vi "Write $GPRMC.vi"(8 "error in (no error)":errorcluster, 10 "GPRMC-data":T1={"TimeStamp"=timestamp(0 s since 1904-01-01), "Validity"=FALSE, "Latitude"=0.0, "Latitude-Direction"=enum."North", "Longitude"=0.0, "Longitude-Direction"=enum."East", "Speed in knots"=0.0, "True course"=0.0, "Date Stamp"=timestamp(0 s since 1904-01-01), "Magnetic Variation (East/West)"=0.0, "GPS Latitude"=0.0, "GPS Longitude"=0.0} {"GPS Longitude" format="%.6f"; "GPS Latitude" format="%.6f"; "Magnetic Variation (East/West)" format="%.02f [deg]"; "Date Stamp" format="%<%x>T"; "True course" format="%.02f [deg]"; "Speed in knots" format="%.02f [kts]"; "Longitude" format="%0.4f [long]"; "Latitude" format="%.04f [lat]"; "TimeStamp" format="%<%.2X>T"}, 11 "GPS Data Message in":refnum<class "GPS Data Message.lvclass">) -> (0 "error out":errorcluster, 3 "GPS Data Message out":refnum<class "GPS Data Message.lvclass">)   [LabVIEW 2015, in "RDS Child Messages.lvlib" / "GPS Data Message.lvclass"]
uses:
  GPS Data Message.lvclass
  3rd Party/NMEA_GPS/NMEA_GPRMC-data.ctl
  3rd Party/NMEA_GPS/NMEA_LatitudeDirection.ctl
  3rd Party/NMEA_GPS/NMEA_LongitudeDirection.ctl
  GPS Data Message.lvclass/GPS Data Message.ctl
  3rd Party/NMEA_GPS/NMEA.lvlib
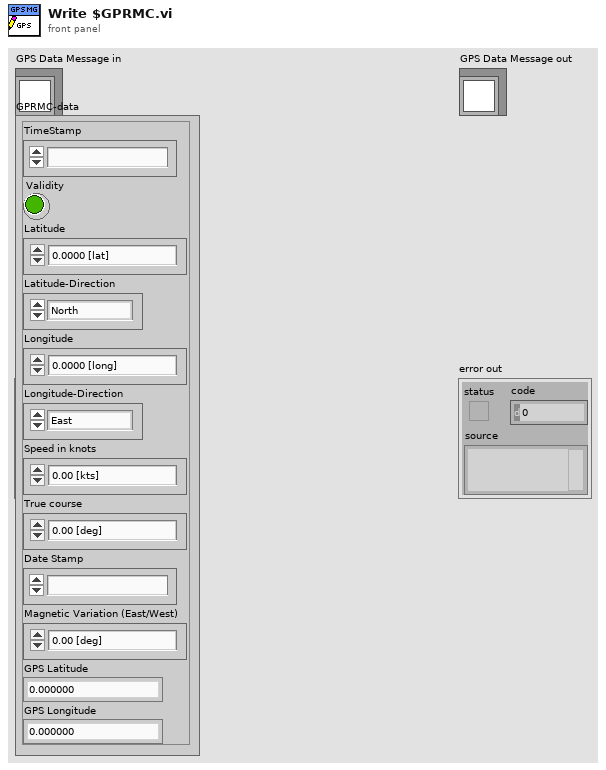
[diagram p1: front panel]
types:
  T1 = typedef "RDS Libraries.lvlib/NMEA.lvlib/NMEA_GPRMC-data.ctl" = cluster{"TimeStamp":timestamp, "Validity":bool, "Latitude":dbl, "Latitude-Direction":T2, "Longitude":dbl, "Longitude-Direction":T3, "Speed in knots":sgl, "True course":sgl, "Date Stamp":timestamp, "Magnetic Variation (East/West)":sgl, "GPS Latitude":dbl, "GPS Longitude":dbl}
  T2 = typedef "RDS Libraries.lvlib/NMEA.lvlib/NMEA_LatitudeDirection.ctl" = enum16{"", "North", "South"}
  T3 = typedef "RDS Libraries.lvlib/NMEA.lvlib/NMEA_LongitudeDirection.ctl" = enum16{"", "East", "West"}
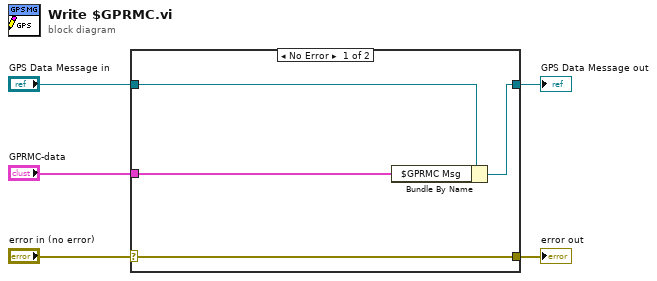
[diagram p0: block diagram]
diagram:
  n1 = case shown="No Error" "error in (no error)" {
    selector: "error in (no error)" -> [w9 w10]
    tunnel: [w9 w10] -> w4
    tunnel: [w7 w11] -> w2
    tunnel: "GPS Data Message in" -> [w8 w11]
    tunnel: "GPRMC-data" -> [w6 _]
    frame No Error {
      n2 = Bundle By Name(cluster=w8, "$GPRMC Msg"=w6) -> (w7:refnum<class "GPS Data Message.lvclass">)
    }
    frame Error {
    }
  }
  "error out" <- w4
  "GPS Data Message out" <- w2
